vi "Untitled 1.vi"() -> ()   [LabVIEW 2021]
uses:
  <instrlib>/Keithley 622x LV 2009/Configure/Display/Typedefs/KE622x -- Display Params.ctl
  <instrlib>/Keithley 622x LV 2009/Configure/Trigger/Typedefs/KE622x -- Arm Layer Params.ctl
  <instrlib>/Keithley 622x LV 2009/Configure/Trigger/Low Level/Typedefs/KE622x -- Arm Source.ctl
  <instrlib>/Keithley 622x LV 2009/Configure/Trigger/Low Level/Typedefs/KE622x -- Trig Link Line.ctl
  <instrlib>/Keithley 622x LV 2009/Configure/Trigger/Low Level/Typedefs/KE622x -- Arm Timer Interval.ctl
  <instrlib>/Keithley 622x LV 2009/Configure/Trigger/Low Level/Typedefs/KE622x -- Arm Output Mode.ctl
  <instrlib>/Keithley 622x LV 2009/Configure/Trigger/Typedefs/KE622x -- Trig Layer Params.ctl
  <instrlib>/Keithley 622x LV 2009/Configure/Trigger/Low Level/Typedefs/KE622x -- Trig Source.ctl
  <instrlib>/Keithley 622x LV 2009/Configure/Trigger/Low Level/Typedefs/KE622x -- Trig Output Mode.ctl
  <instrlib>/Keithley 622x LV 2009/Configure/Source/Typedefs/KE622x -- Sweep Type.ctl
  <instrlib>/Keithley 622x LV 2009/Typedefs/KE622x -- On Off Control.ctl
  <instrlib>/Keithley 622x LV 2009/Configure/Source/Typedefs/KE622x -- List Sweep Params.ctl
  <instrlib>/Keithley 622x LV 2009/Configure/Source/Typedefs/KE622x -- List Sweep Steps.ctl
  <instrlib>/Keithley 622x LV 2009/Configure/Source/Typedefs/KE622x -- List Sweep Step.ctl
  <instrlib>/Keithley 622x LV 2009/Configure/Source/Typedefs/KE622x -- Current Level.ctl
  <instrlib>/Keithley 622x LV 2009/Configure/Source/Typedefs/KE622x -- Source Delay.ctl
  <instrlib>/Keithley 622x LV 2009/Configure/Source/Typedefs/KE622x -- Voltage Limit.ctl
  <instrlib>/Keithley 622x LV 2009/Keithley 622x1.lvlib
panel:
  in  "VISA resource name":refnum<visa-resource-name>
  in  "error in (no error)":errorcluster
  out "error out":errorcluster
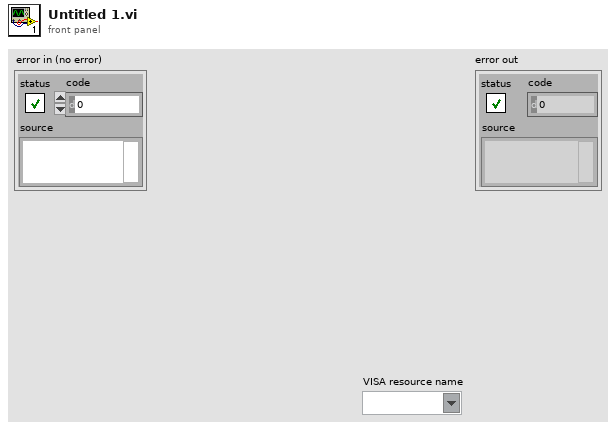
[diagram p1: front panel]
types:
  T1 = typedef "Keithley 622x1.lvlib/KE622x -- List Sweep Params.ctl" = cluster{"Abort On\nCompliance?":bool, "List Sweep Steps":T2}
  T2 = typedef "Keithley 622x1.lvlib/KE622x -- List Sweep Steps.ctl" = T3[]
  T3 = typedef "Keithley 622x1.lvlib/KE622x -- List Sweep Step.ctl" = cluster{"Current Level (A)":T4, "Source Delay (s)":T5, "Voltage Limit (V)":T6}
  T4 = typedef "Keithley 622x1.lvlib/KE622x -- Current Level.ctl" = dbl
  T5 = typedef "Keithley 622x1.lvlib/KE622x -- Source Delay.ctl" = dbl
  T6 = typedef "Keithley 622x1.lvlib/KE622x -- Voltage Limit.ctl" = dbl
  T7 = typedef "Keithley 622x1.lvlib/KE622x -- On Off Control.ctl" = enum16{"Off", "On"}
  T8 = typedef "Keithley 622x1.lvlib/KE622x -- Sweep Type.ctl" = enum16{"Linear", "Log", "List"}
  T9 = typedef "Keithley 622x1.lvlib/KE622x -- Trig Layer Params.ctl" = cluster{"Input Trig Source":T10, "Input Trig Link Line":T11, "Output Trig Mode":T12, "Output Trig Link Line":T11}
  T10 = typedef "Keithley 622x1.lvlib/KE622x -- Trig Source.ctl" = enum16{"Immediate", "Trigger Link"}
  T11 = typedef "Keithley 622x1.lvlib/KE622x -- Trig Link Line.ctl" = enum16{"1", "2", "3", "4", "5", "6"}
  T12 = typedef "Keithley 622x1.lvlib/KE622x -- Trig Output Mode.ctl" = enum16{"No Trig Out", "Source Turn On", "After Source Delay"}
  T13 = typedef "Keithley 622x1.lvlib/KE622x -- Arm Layer Params.ctl" = cluster{"Bypass Arm Layer\nInput Trigger?":bool, "Input Trig Source":T14, "Input Trig Link Line":T11, "Arm Timer Interval (s)":T15, "Output Trig Mode":T16, "Output Trig Link Line":T11}
  T14 = typedef "Keithley 622x1.lvlib/KE622x -- Arm Source.ctl" = enum16{"Immediate", "Bus (*TRG)", "Timer", "Manual", "Trigger Link", "SOT Falling Edge", "SOT Rising Edge", "SOT Either Edge"}
  T15 = typedef "Keithley 622x1.lvlib/KE622x -- Arm Timer Interval.ctl" = dbl
  T16 = typedef "Keithley 622x1.lvlib/KE622x -- Arm Output Mode.ctl" = enum16{"No Trig Out", "Trig Out On Enter Arm", "Trig Out On Exit Arm"}
  T17 = typedef "Keithley 622x1.lvlib/KE622x -- Display Params.ctl" = cluster{"Display\nEnabled?":bool, "Custom Top\nLine Text?":bool, "Top Line Text (20 chars max)":string, "Custom Bottom\nLine Text?":bool, "Bottom Line Text (32 chars max)":string}
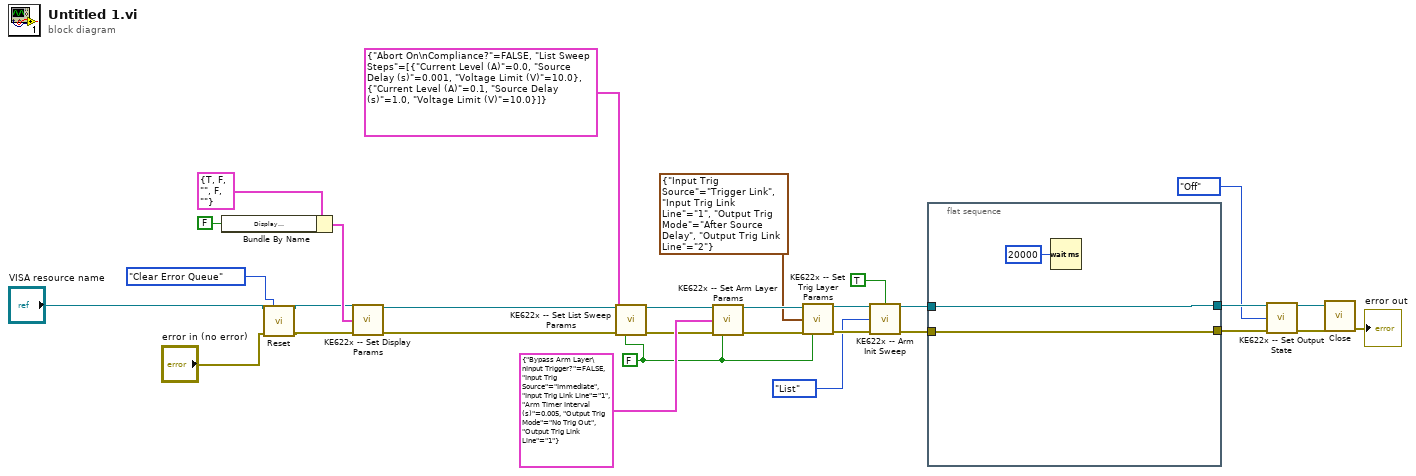
[diagram p0: block diagram]
diagram:
  w11 = FALSE ("Read Back Set Values? (T)")
  n1 = Bundle By Name(cluster=T17 {"Display\nEnabled?"=TRUE, "Custom Top\nLine Text?"=FALSE, "Top Line Text (20 chars max)"="", "Custom Bottom\nLine Text?"=FALSE, "Bottom Line Text (32 chars max)"=""} ("Display Params"), "Display\nEnabled?"=FALSE ("Display\nEnabled?")) -> (w28:T17)
  n2 = call <instrlib>:"Reset.vi"("VISA resource name"="VISA resource name", "Error Queue Option"=enum16{"Clear Error Queue", "Error Query"}."Clear Error Queue", "error in (no error)"="error in (no error)") -> ("VISA resource name out"=w5:refnum<visa-resource-name>, "error out"=w4:errorcluster)  [unwired: 11 in]
  n3 = call <instrlib>:"KE622x -- Set Display Params.vi"("Resource In"=w5, "Display Params"=w28, "error in (no error)"=w4) -> ("Resource Out (dupl)"=w7:refnum<visa-resource-name>, "error out"=w10:errorcluster)  [unwired: 11 in]
  n4 = call <instrlib>:"KE622x -- Set List Sweep Params.vi"("Resource In"=w7, "List Sweep Params In"=T1 {"Abort On\nCompliance?"=FALSE, "List Sweep Steps"=[{"Current Level (A)"=0.0, "Source Delay (s)"=0.001, "Voltage Limit (V)"=10.0}, {"Current Level (A)"=0.1, "Source Delay (s)"=1.0, "Voltage Limit (V)"=10.0}]}, "error in (no error)"=w10, "Read Back Set Values? (T)"=w11) -> ("Resource Out (dupl)"=w8:refnum<visa-resource-name>, "error out"=w9:errorcluster)  [unwired: 9 in, 1 out]
  n5 = call <instrlib>:"KE622x -- Set Arm Layer Params.vi"("Resource In"=w8, "Arm Layer Params In"=T13 {"Bypass Arm Layer\nInput Trigger?"=FALSE, "Input Trig Source"=enum."Immediate", "Input Trig Link Line"=enum."1", "Arm Timer Interval (s)"=0.005, "Output Trig Mode"=enum."No Trig Out", "Output Trig Link Line"=enum."1"}, "error in (no error)"=w9, "Read Back Set Values? (T)"=w11) -> ("Resource Out (dupl)"=w26:refnum<visa-resource-name>, "error out"=w25:errorcluster)  [unwired: 9 in, 1 out]
  n6 = call <instrlib>:"KE622x -- Set Trig Layer Params.vi"("Resource In"=w26, "Trig Layer Params In"=T9 {"Input Trig Source"=enum."Trigger Link", "Input Trig Link Line"=enum."1", "Output Trig Mode"=enum."After Source Delay", "Output Trig Link Line"=enum."2"}, "error in (no error)"=w25, "Read Back Set Values? (T)"=w11) -> ("Resource Out (dupl)"=w23:refnum<visa-resource-name>, "error out"=w22:errorcluster)  [unwired: 9 in, 1 out]
  n7 = call <instrlib>:"KE622x -- Arm Init Sweep.vi"("Resource In"=w23, "Init Sweep? (T)"=TRUE, "Sweep Type"=KE622x_--_Sweep_Type."List", "error in (no error)"=w22) -> ("Resource Out (dupl)"=w20:refnum<visa-resource-name>, "error out"=w19:errorcluster)  [unwired: 10 in]
  n8 = flat-sequence {
    tunnel: w20 -> [w31]
    tunnel: [w32] -> w18
    tunnel: w19 -> [w32]
    tunnel: [w31] -> w17
    frame #0 {
      n9 = Wait (ms)(milliseconds to wait=u32 20000) -> ()  [unwired: 1 out]
    }
  }
  n10 = call <instrlib>:"KE622x -- Set Output State.vi"("Resource In"=w17, "Output State"=KE622x_--_On_Off_Control."Off", "error in (no error)"=w18) -> ("Resource Out (dupl)"=w15:refnum<visa-resource-name>, "error out"=w14:errorcluster)  [unwired: 11 in]
  n11 = call <instrlib>:"Close.vi"("VISA resource name"=w15, "error in (no error)"=w14) -> ("error out"=→"error out":errorcluster)  [unwired: 13 in]
